vi "Database.WriteStationValues.vi"(8 "error in":errorcluster, 10 "FileBody":T1 {"Values" format="%.3f"}, 11 "Data in":T2 {"Variant"."TS"."TV"."minimum" format="%#.3f"; "Variant"."TS"."TV"."maximum" format="%#.3f"; "Variant"."TS"."TP"."value" format="%#.3f"}) -> (0 "error out":errorcluster, 3 "Data out":T2 {"Variant"."TS"."TV"."minimum" format="%#.3f"; "Variant"."TS"."TV"."maximum" format="%#.3f"; "Variant"."TS"."TP"."value" format="%#.3f"})   [LabVIEW 2016]
doc: "Write test results (measurement values) to proda database\n\nWabco 2017 All right reserved\nAuthor: maciej.szupienko@wabco-auto.com"
uses:
  Tools/Translator/Translator.Message.ctl
  Tools/EventLog/EventLog.EventSource.ctl
  Tools/EventLog/EventLog.New(array).vi
  Database.Main.Data.Sets.ctl
  Database.Main.Data.Status.ctl
  ProdaNG/Controls/ProdaNG.ProcessResult.ctl
  ProdaNG/Controls/ProdaNG.ProcessStepResult.ctl
  ProdaNG/Controls/ProdaNG.TestStepResult.ctl
  ProdaNG/Controls/ProdaNG.TestValueResult.ctl
  ProdaNG/Controls/ProdaNG.Identification.ctl
  Database.Main.Data.ctl
  Database.Main.Data.Results.ctl
  ProdaNG/Controls/ProdaNG.TestStepParam.ctl
  ProdaNG/Controls/ProdaNG.TestValue.ctl
  ProdaNG/Controls/ProdaNG.TestStep.ctl
  ProdaNG/Controls/ProdaNG.ProcessStepParam.ctl
  Database.Main.Data.Variant.ctl
  Logger/Logger.FileBody.ctl
panel:
  out "Prod saved":bool
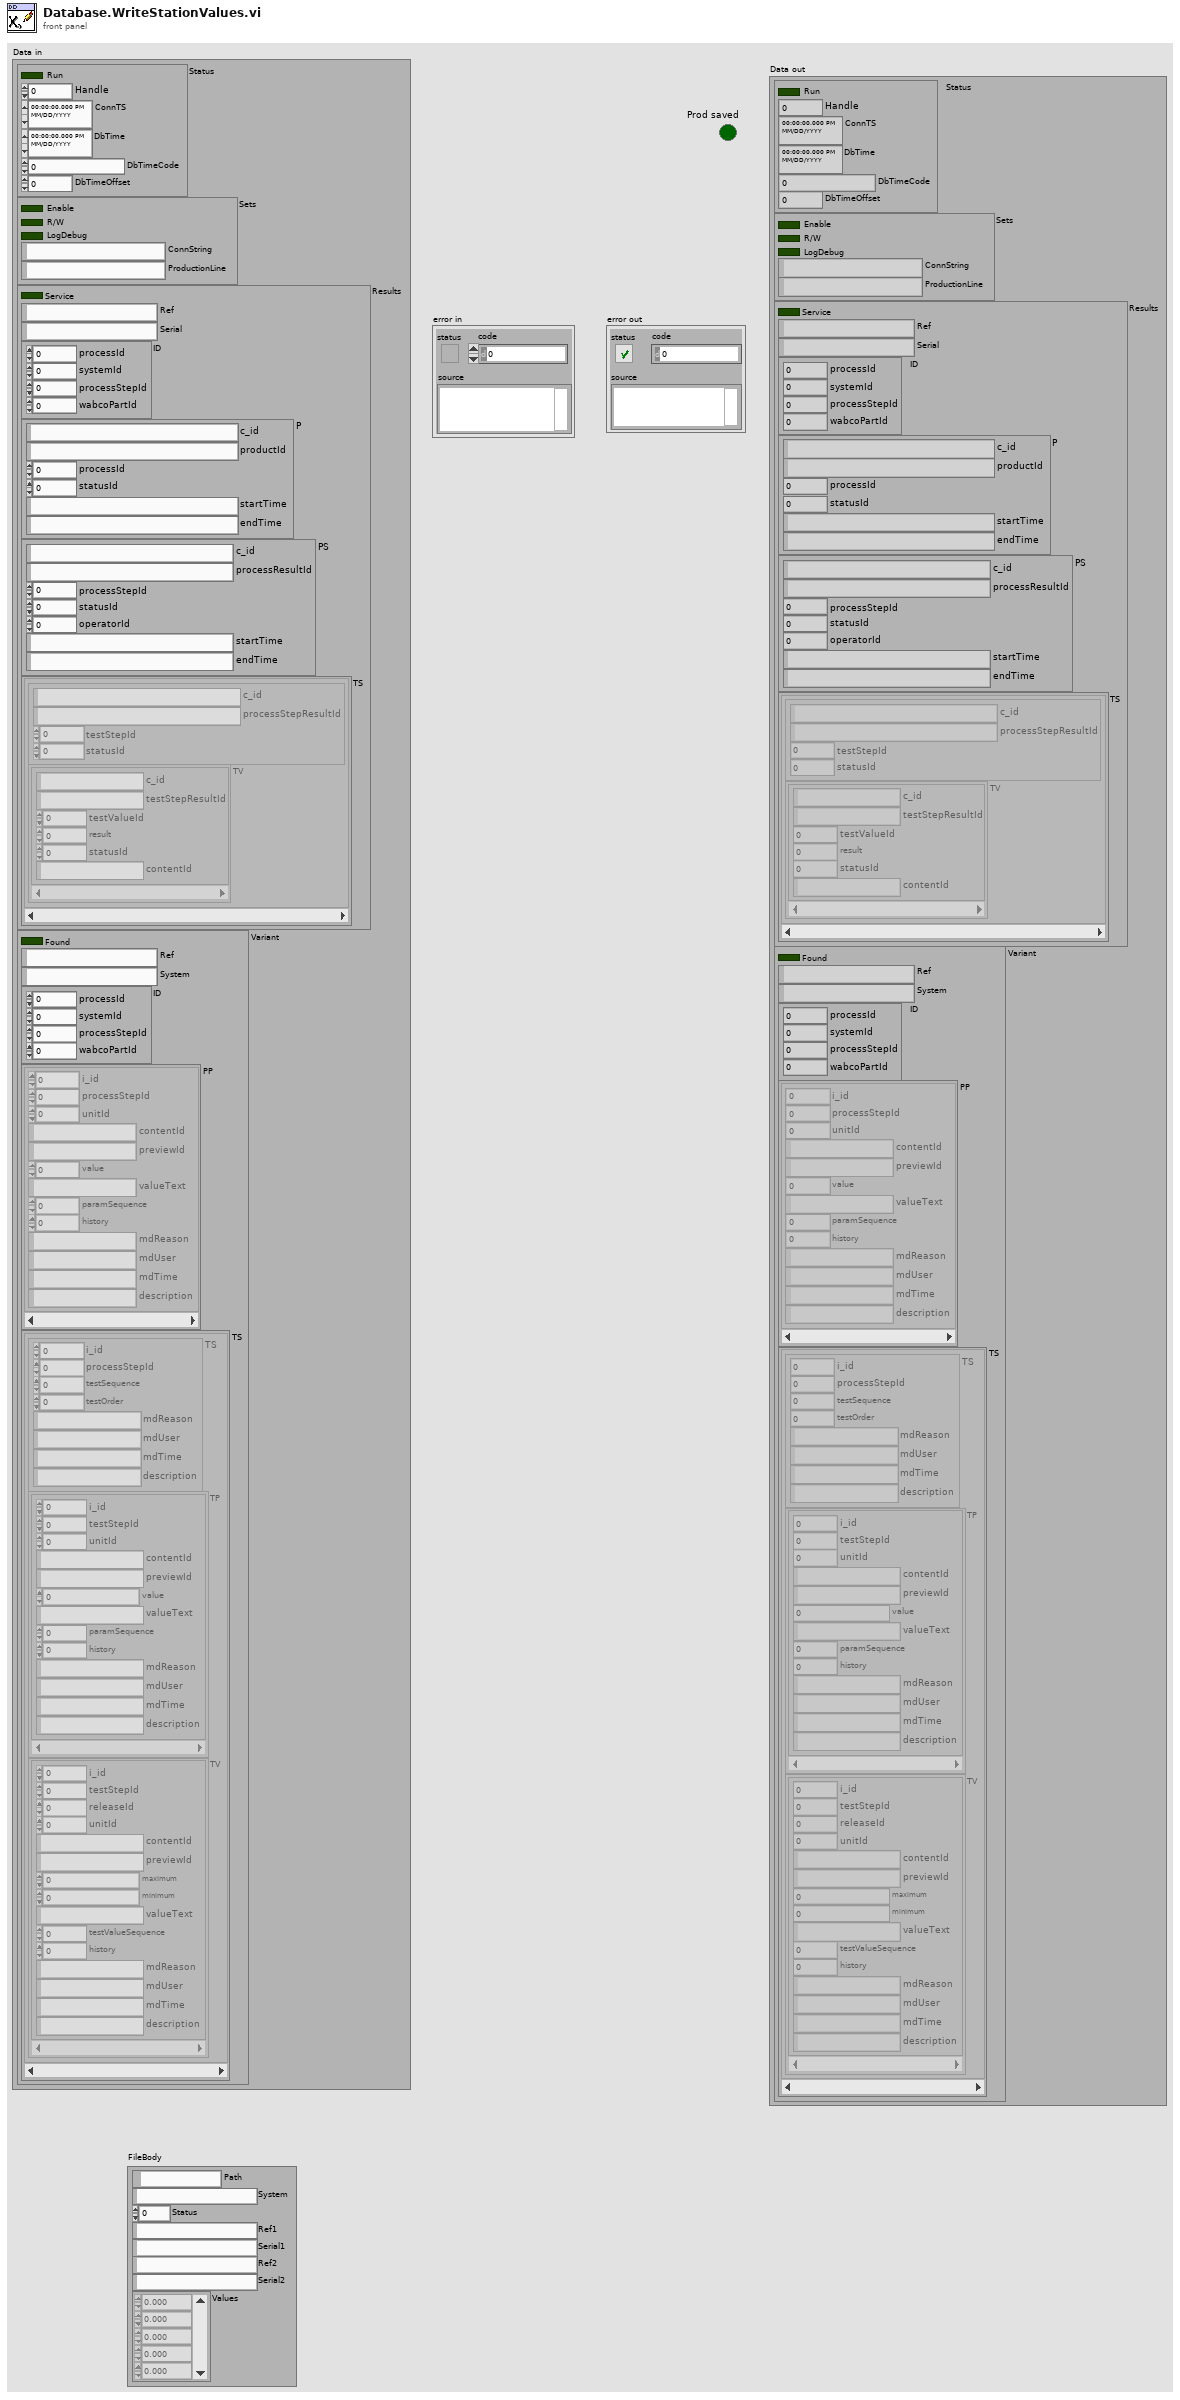
[diagram p1: front panel]
types:
  T1 = typedef "Logger.FileBody.ctl" = cluster{"Path":path, "System":string, "Status":u8, "Ref1":string, "Serial1":string, "Ref2":string, "Serial2":string, "Values":sgl[]}
  T2 = typedef "Database.Main.Data.ctl" = cluster{"Status":T3, "Sets":T4, "Results":T5, "Variant":T11}
  T3 = typedef "Database.Main.Data.Status.ctl" = cluster{"Run":bool, "Handle":i32, "ConnTS":timestamp, "DbTime":timestamp, "DbTimeCode":dbl, "DbTimeOffset":dbl}
  T4 = typedef "Database.Main.Data.Sets.ctl" = cluster{"Enable":bool, "R/W":bool, "LogDebug":bool, "ConnString":string, "ProductionLine":string}
  T5 = typedef "Database.Main.Data.Results.ctl" = cluster{"Service":bool, "Ref":string, "Serial":string, "ID":T6, "P":T7, "PS":T8, "TS":cluster{"TS":T9, "TV":T10[]}[]}
  T6 = typedef "ProdaNG.Identification.ctl" = cluster{"processId":i32, "systemId":i32, "processStepId":i32, "wabcoPartId":i32}
  T7 = typedef "ProdaNG.ProcessResult.ctl" = cluster{"c_id":string, "productId":string, "processId":i32, "statusId":i32, "startTime":string, "endTime":string}
  T8 = typedef "ProdaNG.ProcessStepResult.ctl" = cluster{"c_id":string, "processResultId":string, "processStepId":i32, "statusId":i32, "operatorId":i32, "startTime":string, "endTime":string}
  T9 = typedef "ProdaNG.TestStepResult.ctl" = cluster{"c_id":string, "processStepResultId":string, "testStepId":i32, "statusId":i32}
  T10 = typedef "ProdaNG.TestValueResult.ctl" = cluster{"c_id":string, "testStepResultId":string, "testValueId":i32, "result":dbl, "statusId":i32, "contentId":string}
  T11 = typedef "Database.Main.Data.Variant.ctl" = cluster{"Found":bool, "Ref":string, "System":string, "ID":T6, "PP":T12[], "TS":cluster{"TS":T13, "TP":T14[], "TV":T15[]}[]}
  T12 = typedef "ProdaNG.ProcessStepParam.ctl" = cluster{"i_id":i32, "processStepId":i32, "unitId":i32, "contentId":string, "previewId":string, "value":dbl, "valueText":string, "paramSequence":i32, "history":i32, "mdReason":string, "mdUser":string, "mdTime":string, "description":string}
  T13 = typedef "ProdaNG.TestStep.ctl" = cluster{"i_id":i32, "processStepId":i32, "testSequence":i32, "testOrder":i32, "mdReason":string, "mdUser":string, "mdTime":string, "description":string}
  T14 = typedef "ProdaNG.TestStepParam.ctl" = cluster{"i_id":i32, "testStepId":i32, "unitId":i32, "contentId":string, "previewId":string, "value":dbl, "valueText":string, "paramSequence":i32, "history":i32, "mdReason":string, "mdUser":string, "mdTime":string, "description":string}
  T15 = typedef "ProdaNG.TestValue.ctl" = cluster{"i_id":i32, "testStepId":i32, "releaseId":i32, "unitId":i32, "contentId":string, "previewId":string, "maximum":dbl, "minimum":dbl, "valueText":string, "testValueSequence":i32, "history":i32, "mdReason":string, "mdUser":string, "mdTime":string, "description":string}
  T16 = typedef "EventLog.EventSource.ctl" = enum16{"All", "Gui", "Cache", "PLC1", "PLC2", "PLC3", "DB", "DB01", "DB02", "DB03", "DB04", "DB05", "DB06", "DB07", "DB08", "DB09", "DB10", "DB11", "DB12", "DB13", "DB14", "DB15", "DB16"}
  T17 = typedef "Translator.Message.ctl" = enum16{"-", "Event confirmed", "Log out", "Log in", "Shutdown", "Cancel", "Start", "Begin time", "End time", "Duration", "Service Mode", "Ignore Results", "Serial Format", "On", "Off", "OK", "NOK", "NOK %s", "Home", "Work", "Close", "Open", "In progress...", "Missing", "Empty", "Hardware failure", "Initial", "Default", "Total", "Out of range", "Free disk space is below 1GB - contact technician", "Error %d >> %s", "Error %d >> %s >> %s", "Msg %d >> %s", "Laser msg %d %s", "Laser cmd error %s %d", "Laser cmd failed %s", "Laser cmd warning %s", "Laser disconnected", "Laser status %s", "Laser already started", "Laser job unkonwn %s", "Laser job missing %s", "Laser job select failure %s", "Unable to start laser printing (%s)", "Unable to stop laser printing (%s)", "Laser marking aborted", "Laser marking timeout", "Unable to reset Laser Interlock (%s)", "Unable to trigger Laser. Laser not ready (%s)", "Laser job '%s' coordinates not configured", "Starting %s", "Quitting %s", "Configured", "Initializing", "Quitting", "Loading", "Loaded %d results", "Loaded %d events", "Running", "Stopped", "Summary", "Laser", "Do you want to continue?", "Do you want to delete the configuration?", "The configuration is being used by an order. Unable to delete!", "Press confirm button", "Station is not based. Do you want to exit?", "Station requires changeover. Do you want to run the test?", "Test options are not set as default. Do you want to continue?", "Formatting of WabcoNo is disabled. Do you want to continue?", "Product not detected. Do you want to continue?", "Product scan failed. Do you want to continue?", "Calibration", "Log out?", "System", "All", "IDLE", "Translating...%s", "Not found", "Alarm %s", "Run", "Skip", "Abort", "Repeat", "Please wait...", "Database disconnected", "Database disconnected - changeover disabled!", "Login to database successful", "Login to database failed: %d; %s", "Unable to check the product status of reference %d - database disconnected", "Unable to set the product status of reference %d - database disconnected", "Variant file backup %s", "Read variant (%s)", "Result", "Station armed!", "Station requires changeover!", "Select reference number...", "EMERGENCY BUTTON - press Control button", "EMERGENCY DOOR - press Control button", "Resetting Emergency...", "Unable to reset safety circuit - Emergency Button pressed", "Unable to reset safety circuit - Emergency Side Door open", "Station not based", "Station based", "Station not empty", "Station basing...", "No order", "Press Start to begin new order", "Scanning new order", "Order NOK. Correct or scan again", "Order OK. Press Accept", "Order ready", "Revolver incorrect", "Fork incorrect", "Revolver missing", "Revolver empty", "Container missing", "Offline results", "Offline statistics", "Updating statistics %.1f %%", "DMC Configurator", "Door open", "Close the front door", "Press start button", "Done. Open the front door", "Running...", "Running...%.1f %%", "Pause %s", "Pause %s. NOK container missing", "Pause %s. OK container missing", "Pause %s. Revolver empty", "Pause %s. Revolver missing", "Pause %s. Revolver incorrect", "Pause %s. Fork missing", "Pause %s. Fork incorrect", "Pause %s. Too many failures", "Pause %s. Unloading failure", "Pause %s. One slot is not working", "Pause %s. Part order is done. Empty OK container", "Pause %s. Unable to move product to slot", "Pause %s. Unable to move back product pusher", "Pause %s. Unable to lift product", "Pause %s. Unable to move back product lifter", "Pause %s. Unable to move product arm to Work", "Pause %s. Unable to move product arm to NOK", "Pause %s. Unable to move product arm to OK", "Pause %s. Unable to unsuck the NOK product", "Pause %s. Unable to drop the NOK product", "Pause %s. Product OK missing", "Pause %s. Unable to unsuck the OK product", "Pause %s. Unable to drop the OK product", "Stopping...", "File '%s' is missing", "File '%s' is broken", "File '%s' is running", "Log file started (%s)", "Log file ended (%s)", "Log file stopped (%s)", "Log file ignored (%s)", "Log file exported (%s)", "Log file export failed (%s)", "Wrong serial number in log file", "Wrong reference number in log file", "Test steps are missing", "%s = %.3f", "Process param '%s' not found in DB", "Process param '%s' wrong order", "Process param '%s' value %.3f out of limits (%.3f; %.3f)", "Step%d param '%s' not found in DB", "Step%d param '%s' wrong order", "Step%d param '%s' value %.3f out of limits (%.3f; %.3f)", "Step%d EV '%s' not found in DB", "Step%d EV '%s' wrong order", "\"%s\" not found in DB", "\"%s\" wrong order", "\"%s\" value %.3f out of limits (%.3f; %.3f)", "\"%s\" not found in software", "Process init (%s)", "Process started", "Process restarted", "Process run", "Process done", "Process done - remove OK container", "Process aborted", "Process aborted at work", "Process aborted at home", "Process error", "Process error at home", "Process error at work", "Process close", "Process pause", "Process continue", "Process door open", "Process door close", "Process pause at slot %s due to %s", "Select plate from the order to process", "Do you want to start the process?", "Do you want to continue the process?", "There is unfinished order. Do you want to put the new order?", "Product %s %d OK", "Product %s %d NOK", "Unable to unload the slot %s. Product missing in the slot", "Unable to unload the slot %s. Product already in the arm", "Unable to accept the product as OK. Product missing in slot %s", "Unable to accept the product as OK. Product could not drop into the container at slot %s", "Unable to accept the product as NOK. Product could not drop into the container at slot %s", "Scan failed. Error %s", "Scan failed. Scanner disconnected", "Scan failed. Wrong Wabco number %d, limit (%d,%d)", "Scan failed. Wrong serial number %d, limit (%d,%d)", "Scan failed. Wrong date %d, limit (%d,%d)", "Scan failed. Wrong product wabco number %d (expected %d)", "Scan failed. Wrong product serial number %d (expected > 0)", "Scan OK %s", "Scan failed. Unable to determine table position (%s)", "Scan failed. Timeout", "Tune failed. Scanner disconnected", "Tune failed. Timeout", "%s = %d", "%s = %d->%d", "Unable to set %s = %.2f - Air Pressure Inside off", "Unable to set digital output '%s' = %d", "Unable to activate air pressure inside - timeout", "Unable to activate air pressure inside - aborted", "Unable to switch on Air Main Valve - Air Pressure Inlet off", "Unable to switch on Air Main Valve - Door open", "Unable to switch off Air Main Valve - timeout", "Unable to switch off Air Main Valve - aborted", "Unable to rotate Table - timeout", "Unable to rotate Table - aborted", "Unable to rotate Table - Product Move not in Home position", "Unable to rotate Table - Air Pressure Inside off", "Unable to rotate Table - Product Lift A not in Home position", "Unable to rotate Table - Product Lift B not in Home position", "Unable to rotate Table - unlock before movement timeout", "Unable to rotate Table - lock after movement timeout", "Unable to move Table Lock to %s position - timeout", "Unable to move Table Lock to %s position - aborted", "Unable to move Table Lock to %s position - Air Pressure Inside off", "Unable to move Table Lock to %s position - Table not in position", "Unable to move Product Lift A to %s position - timeout", "Unable to move Product Lift B to %s position - timeout", "Unable to move Product Lift A to %s position - aborted", "Unable to move Product Lift B to %s position - aborted", "Unable to move Product Lift A to %s position - Air Pressure Inside off", "Unable to move Product Lift B to %s position - Air Pressure Inside off", "Unable to move Product Lift A to %s position - Table not locked", "Unable to move Product Lift B to %s position - Table not locked", "Unable to move Product Lift A to %s position - Product Arm not in Work position", "Unable to move Product Lift B to %s position - Product Arm not in Work position", "Unable to set Product Suction Gripper %s to %s - timeout", "Unable to set Product Suction Gripper %s to %s - aborted", "Unable to set Product Suction Gripper %s to %s - Air Pressure Inside off", "Unable to set Product Suction Gripper %s to %s - Table slot unkown", "Unable to move Product Arm to %s position - timeout", "Unable to move Product Arm to %s position - aborted", "Unable to move Product Arm to %s position - Air Pressure Inside off", "Unable to move Product Arm to %s position - Product Lift A not in Home position", "Unable to move Product Arm to %s position - Product Lift B not in Home position", "Unable to move Product to %s position - timeout", "Unable to move Product to %s position - aborted", "Unable to move Product to %s position - Air Pressure Inside off", "Unable to move Product to %s position - Table not in position"}
  T18 = typedef "ProdaNG.Product.ctl" = cluster{"c_id":string, "wabcoPartId":i32, "serialNumber":string, "comment":string, "individual":i32, "crProcessStepId":i32, "mdProcessStepId":i32, "crTime":string, "mdTime":string}
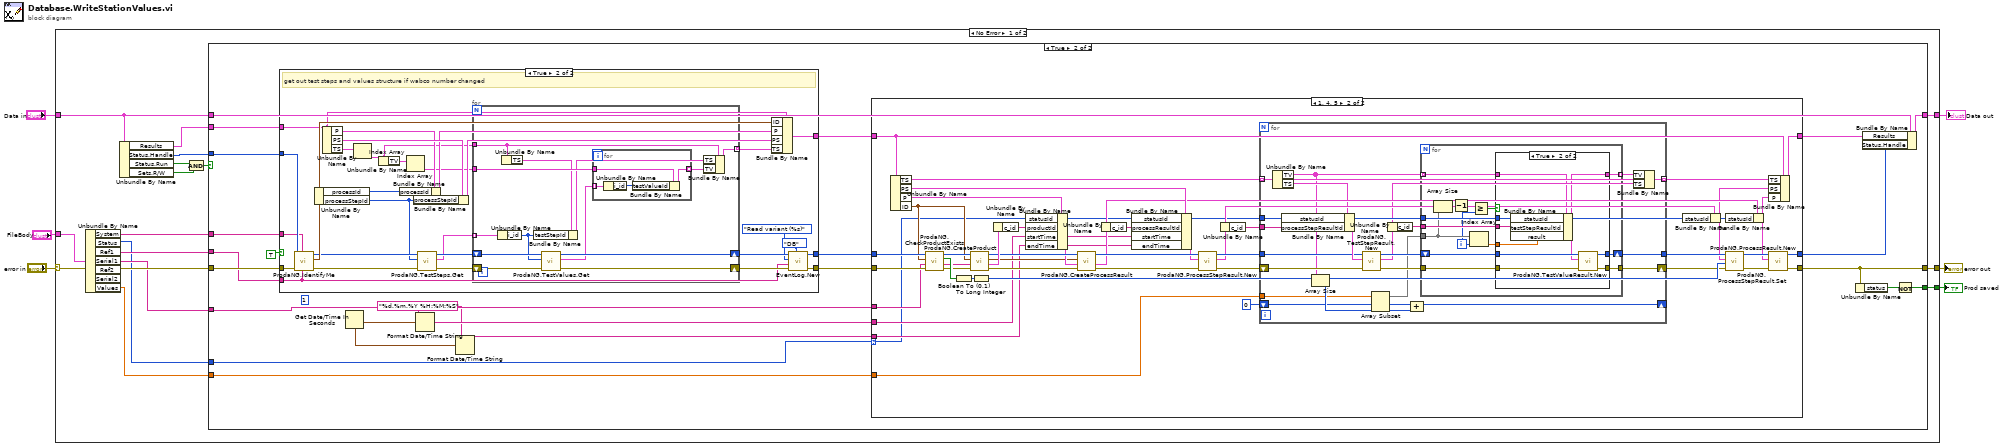
[diagram p0: block diagram]
diagram:
  n1 = case shown="No Error" "error in" {
    selector: "error in" -> [w11 w189]
    tunnel: [w18 w189] -> w6
    tunnel: "Data in" -> [w21 w188]
    tunnel: [w20 w188] -> w3
    tunnel: [w16 _] -> w2
    tunnel: "FileBody" -> [w13 _]
    frame No Error {
      n2 = Unbundle By Name(w13) -> ("System"=w12:string, "Status"=w8:u8, "Ref1"=w10:string, "Serial1"=w9:string, "Values"=w7:sgl[])  [unwired: 2 out]
      n3 = Unbundle By Name(w21) -> ("Results"=w19:T5, "Status.Handle"=w22:i32, "Status.Run"=w17:bool, "Sets.R/W"=w14:bool)
      n4 = Compound Arithmetic op=AND(w17, w14) -> (w15:bool)
      n5 = case shown="True" w15 {
        tunnel: w11 -> [w24 w47]
        tunnel: w22 -> [_ w46]
        tunnel: w21 -> [w23 w45]
        tunnel: [w23 w44] -> w20
        tunnel: w19 -> [_ w43]
        tunnel: [w24 w25] -> w18
        tunnel: [_ w35] -> w16
        tunnel: w12 -> [_ w34]
        tunnel: w10 -> [_ w33]
        tunnel: w9 -> [_ w32]
        tunnel: w8 -> [_ w29]
        tunnel: w7 -> [_ w26]
        frame False {
        }
        frame True {
          w28 = "%d.%m.%Y %H:%M:%S" ("time format string (%c)")
          (unwired) 1
          n6 = case shown="True" TRUE {
            tunnel: w33 -> [_ w154]
            tunnel: w47 -> [w142 w160]
            tunnel: [w142 w157] -> w42
            tunnel: w46 -> [w141 w159]
            tunnel: [w141 w153] -> w41
            tunnel: w43 -> [w140 w151]
            tunnel: [w140 w158] -> w37
            tunnel: w34 -> [_ w143]
            frame False {
            }
            frame True {
              # "get out test steps and values structure if wabco number changed"
              n7 = call "ProdaNG.IdentifyMe.vi"("wabcoNumber"=w154, "systemName"=w143, "error in"=w160, "dbHandleIn"=w159) -> ("error out"=w161:errorcluster, "Identification"=w169:T6, "dbHandle"=w162:i32)  [unwired: 5 in]
              n8 = Unbundle By Name(w169) -> ("processId"=w164:i32, "processStepId"=w150:i32)
              n9 = Unbundle By Name(w151) -> ("P"=w167:T7, "PS"=w168:T8, "TS"=w148:cluster{"TS":T9, "TV":T10[]}[])
              n10 = Index Array(array=w148) -> (element=w145:cluster{"TS":T9, "TV":T10[]})  [unwired: 1 in]
              n11 = Unbundle By Name(w145) -> ("TV"=w147:T10[])
              n12 = Bundle By Name(cluster=w167, "processId"=w164) -> (w165:T7)
              n13 = Index Array(array=w147) -> (element=w146:T10)  [unwired: 1 in]
              n14 = Bundle By Name(cluster=w168, "processStepId"=w150) -> (w166:T8)
              n15 = call "ProdaNG.TestSteps.Get.vi"("error in (no error)"=w161, "processStepId"=w150, "dbHandleIn"=w162) -> ("error out"=w163:errorcluster, "TestSteps"=w149:T13[], "dbHandle"=w170:i32)  [unwired: 6 in]
              n16 = for {
                tunnel: w149 -> [w178] mode=indexing
                tunnel: w146 -> [w176]
                shift-right: [w180] -> w153
                shift-left: w170 -> [w183]
                shift-right: [w181] -> w156
                shift-left: w163 -> [w182]
                tunnel: w145 -> [w174]
                tunnel: [w171] -> w144 mode=indexing
                n17 = Unbundle By Name(w178) -> ("i_id"=w177:i32)
                n18 = Unbundle By Name(w174) -> ("TS"=w173:T9)
                n19 = Bundle By Name(cluster=w173, "testStepId"=w177) -> (w172:T9)
                n20 = call "ProdaNG.TestValues.Get.vi"("error in (no error)"=w182, "testStepId"=w177, "dbHandleIn"=w183) -> ("error out"=w181:errorcluster, "TestStepValues"=w179:T15[], "dbHandle"=w180:i32)  [unwired: 6 in]
                n21 = for {
                  tunnel: w179 -> [w187] mode=indexing
                  tunnel: w176 -> [w185]
                  tunnel: [w184] -> w175 mode=indexing
                  n22 = Unbundle By Name(w187) -> ("i_id"=w186:i32)
                  n23 = Bundle By Name(cluster=w185, "testValueId"=w186) -> (w184:T10)
                }
                n24 = Bundle By Name(cluster=w174, "TS"=w172, "TV"=w175) -> (w171:cluster{"TS":T9, "TV":T10[]})
              }
              n25 = Bundle By Name(cluster=w151, "ID"=w169, "P"=w165, "PS"=w166, "TS"=w144) -> (w158:T5)
              n26 = call-poly "EventLog.New.vi"("Source (All)"=EventLog.EventSource."DB", "error in (no error)"=w156, "Arguments"=w154, "Message (-)"=Translator.Message."Read variant (%s)") -> ("error out"=w157:errorcluster)  [unwired: 6 in, 1 out]
            }
          }
          n27 = Get Date/Time In Seconds() -> (seconds since 1Jan1904=w27:timestamp)
          n28 = Format Date/Time String(time format string (%c)=w28, seconds (now)=w27) -> (date/time string=w31:string)  [unwired: 1 in]
          n29 = Format Date/Time String(time format string (%c)=w28, seconds (now)=w27) -> (date/time string=w30:string)  [unwired: 1 in]
          n30 = case shown="1, 4, 5" w29 {
            selector: w29 -> [_ w51]
            tunnel: w42 -> [w50 w72]
            tunnel: w41 -> [w49 w71]
            tunnel: [w48 w63] -> w39
            tunnel: [w49 w59] -> w38
            tunnel: w37 -> [w48 w58]
            tunnel: [w50 w57] -> w25
            tunnel: w32 -> [_ w53]
            tunnel: w30 -> [_ w54]
            tunnel: w31 -> [_ w55]
            tunnel: w26 -> [_ w52]
            frame Default {
            }
            frame 1, 4, 5 {
              n31 = Unbundle By Name(w58) -> ("TS"=w69:cluster{"TS":T9, "TV":T10[]}[], "PS"=w68:T8, "P"=w67:T7, "ID"=w66:T6)
              n32 = call "ProdaNG.CheckProductExists.vi"("error in (no error)"=w72, "serialNumber"=w53, "ID"=w66, "dbHandle"=w71) -> ("error out"=w74:errorcluster, "Results exist?"=w92:bool, "dbHandle out"=w70:i32)  [unwired: 2 in, 3 out]
              n33 = Boolean To (0,1)(Boolean=w92) -> (0, 1=w73:i16)
              n34 = call "ProdaNG.CreateProduct.vi"("error in (no error)"=w74, "serialNumber"=w53, "ID"=w66, "dbHandle"=w70) -> ("error out"=w86:errorcluster, "Product out"=w91:T18, "dbHandle out"=w87:i32)  [unwired: 4 in, 1 out]
              n35 = To Long Integer(number=w73) -> (32bit integer=w90:i32)
              n36 = Unbundle By Name(w91) -> ("c_id"=w77:string)
              n37 = Bundle By Name(cluster=w67, "statusId"=w51, "productId"=w77, "startTime"=w55, "endTime"=w54) -> (w85:T7)
              n38 = call "ProdaNG.CreateProcessResult.vi"("error in (no error)"=w86, "ProcessResult"=w85, "ID"=w66, "dbHandle"=w87) -> ("error out"=w88:errorcluster, "ProcessResult 2"=w64:T7, "dbHandle out"=w89:i32)  [unwired: 5 in]
              n39 = Unbundle By Name(w64) -> ("c_id"=w78:string)
              n40 = Bundle By Name(cluster=w68, "statusId"=w51, "processResultId"=w78, "startTime"=w55, "endTime"=w54) -> (w84:T8)
              n41 = call "ProdaNG.ProcessStepResult.New.vi"("error in (no error)"=w88, "ProcessStepResult"=w84, "dbHandle"=w89) -> ("error out"=w76:errorcluster, "ProcessStepResult out"=w61:T8, "dbHandle"=w75:i32)  [unwired: 6 in]
              n42 = Unbundle By Name(w61) -> ("c_id"=w79:string)
              n43 = for {
                tunnel: [w112] -> w81
                tunnel: w79 -> [w110]
                tunnel: w75 -> [w108]
                tunnel: w69 -> [w103] mode=indexing
                tunnel: w51 -> [w104]
                tunnel: [w99] -> w65 mode=indexing
                shift-right: [w111] -> w80
                shift-left: w76 -> [w109]
                shift-right: [w94] -> _
                shift-left: 0 -> [w96]
                tunnel: w52 -> [w93]
                n44 = Unbundle By Name(w103) -> ("TV"=w98:T10[], "TS"=w101:T9)
                n45 = Bundle By Name(cluster=w101, "statusId"=w104, "processStepResultId"=w110) -> (w113:T9)
                n46 = Array Size(array=w98) -> (size(s)=w97:i32)
                n47 = call "ProdaNG.TestStepResult.New.vi"("error in (no error)"=w109, "TestStepResult"=w113, "dbHandle"=w108) -> ("error out"=w105:errorcluster, "TestStepResult out"=w100:T9, "dbHandle"=w106:i32)  [unwired: 6 in]
                n48 = Array Subset(array=w93, index=w96, length=w97) -> (w95:sgl[])
                n49 = Unbundle By Name(w100) -> ("c_id"=w107:string)
                n50 = Compound Arithmetic op=ADD(w96, w97) -> (w94:i32)
                n51 = for "results" {
                  tunnel: w105 -> [w127]
                  tunnel: [w124] -> w111
                  tunnel: w107 -> [w125]
                  shift-right: [w123] -> w112
                  shift-left: w106 -> [w126]
                  tunnel: w95 -> [w118]
                  tunnel: w104 -> [w122]
                  tunnel: w98 -> [w121] mode=indexing
                  tunnel: [w120] -> w102 mode=indexing
                  i -> [w116]
                  n52 = Array Size(array=w118) -> (size(s)=w115:i32)
                  n53 = Decrement(x=w115) -> (x-1=w114:i32)
                  n54 = Index Array(array=w118, index=w116) -> (element=w119:sgl)
                  n55 = Greater Or Equal?(x=w114, y=w116) -> (x >= y?=w117:bool)
                  n56 = case shown="True" w117 {
                    tunnel: w127 -> [w129 w139]
                    tunnel: w126 -> [w128 w138]
                    tunnel: w125 -> [_ w137]
                    tunnel: [w129 w136] -> w124
                    tunnel: [w128 w135] -> w123
                    tunnel: w122 -> [_ w134]
                    tunnel: w121 -> [w130 w133]
                    tunnel: [w130 w132] -> w120
                    tunnel: w119 -> [_ w131]
                    frame False {
                    }
                    frame True {
                      n57 = Bundle By Name(cluster=w133, "statusId"=w134, "testStepResultId"=w137, "result"=w131) -> (w132:T10)
                      n58 = call "ProdaNG.TestValueResult.New.vi"("error in (no error)"=w139, "TestValueResult"=w132, "dbHandle"=w138) -> ("error out"=w136:errorcluster, "dbHandle"=w135:i32)  [unwired: 7 in]
                    }
                  }
                }
                n59 = Bundle By Name(cluster=w103, "TV"=w102, "TS"=w100) -> (w99:cluster{"TS":T9, "TV":T10[]})
              }
              n60 = Bundle By Name(cluster=w61, "statusId"=w51) -> (w60:T8)
              n61 = call "ProdaNG.ProcessStepResult.Set.vi"("error in (no error)"=w80, "isRepeat (0)"=w90, "ProcessStepResult"=w60, "dbHandle"=w81) -> ("error out"=w83:errorcluster, "dbHandle"=w82:i32)  [unwired: 6 in]
              n62 = Bundle By Name(cluster=w64, "statusId"=w51) -> (w62:T7)
              n63 = Bundle By Name(cluster=w58, "TS"=w65, "PS"=w60, "P"=w62) -> (w63:T5)
              n64 = call "ProdaNG.ProcessResult.New.vi"("error in (no error)"=w83, "ProcessResult"=w62, "dbHandle"=w82) -> ("error out"=w57:errorcluster, "dbHandle"=w59:i32)  [unwired: 6 in, 1 out]
            }
          }
          n65 = Unbundle By Name(w25) -> ("status"=w36:bool)
          n66 = Bundle By Name(cluster=w45, "Results"=w39, "Status.Handle"=w38) -> (w44:T2)
          n67 = Not(x=w36) -> (.not. x?=w35:bool)
        }
      }
    }
    frame Error {
    }
  }
  "error out" <- w6
  "Prod saved" <- w2
  "Data out" <- w3
